vi "Main.vi"(11 "Module Admin":refnum<class "Delacor_lib_QMH_Module Admin.lvclass">) -> ()   [LabVIEW 2016, in "Lab Streaming Layer.lvlib"]
doc: "This template is based off of the Queued Message Handler design pattern and the Queued Message Handler project template that ships with LabVIEW.\n\nThe main difference is that the queue is private to this module and communication between modules is performed via Broadcast and Request events.\n\nRequest events are wrapped in public API methods and are handled in the Event Handling Loop (EHL) of this VI. Any module can register for Broadcast events sent by this module. The EHL generates messages based on user interface actions.\n\nThe Message Handling Loop (MHL) processes messages generated by the EHL, or by other messages. The messages are string values, so new messages can be added easily to the Message Cases case structure in the MHL. Each message cluster can also provide an optional value for Message Data, which is a variant that can be converted to whatever message-specific data is required.\n_____\nBased on DQMH Project Template 7.0.0.1280."
uses:
  Lab Streaming Layer.lvlib
  <vilib>/Delacor/Delacor QMH/Libraries/Module Admin_class/Delacor_lib_QMH_Module Admin.lvclass
  Module Data--cluster.ctl
  Custom Controls/lsl_channel_format.ctl
  Custom Controls/lsl_outlet.ctl
  Custom Controls/lsl_streaminfo.ctl
  Custom Controls/lsl_xml_ptr.ctl
  <vilib>/Delacor/Delacor QMH/Libraries/Message Queue_class/Delacor_lib_QMH_Message Queue.lvclass/Delacor_lib_QMH_Message Queue.ctl
  Stop Argument--cluster.ctl
  <vilib>/Delacor/Delacor QMH/Libraries/Module Admin_class/Delacor_lib_QMH_Module Admin.lvclass/Delacor_lib_QMH_Module Admin.ctl
  Init LSL Metadata Argument--cluster.ctl
  Stop Stream Argument--cluster.ctl
  LSL Stream Data Argument--cluster.ctl
  Acquisition/WiBCI16T_Data.ctl
  Acquisition/WiBCI16T_Status.ctl
  Acquisition/Reg_Map.ctl
  Get Listeners count Argument--cluster.ctl
  Get Listeners count (Reply Payload)--cluster.ctl
  KeyBoard Trigger Argument--cluster.ctl
  <vilib>/Utility/miscctls.llb/LVPointTypeDef.ctl
  <vilib>/Delacor/Delacor QMH/Libraries/Message Queue_class/Delacor_lib_QMH_Enqueue Message (Single).vi
  <vilib>/Delacor/Delacor QMH/Libraries/Module Admin_class/Delacor_lib_QMH_Get External Launch.vi
  <vilib>/Delacor/Delacor QMH/Libraries/Message Queue_class/Delacor_lib_QMH_Message Queue.lvclass
  Settings Editor/Settings Editor.lvlib
  Acquisition/Acquisition.lvlib
panel:
  out "error out 2":errorcluster
  out "error out":errorcluster
  out "Status":string
  in  "Simulate MHL Error":bool
  in  "Simulate EHL Error":bool
  # "This template is for the DQMH framework. See the block diagram for more information on how to use this template."
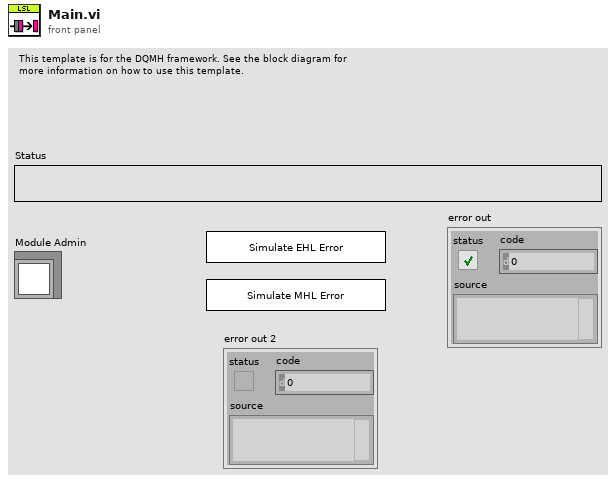
[diagram p1: front panel]
types:
  T1 = typedef "Settings Editor.lvlib/Broadcast Events--cluster.ctl" = cluster{"Module Did Init":refnum<user-event>, "Status Updated":refnum<user-event>, "Error Reported":refnum<user-event>, "Module Did Stop":refnum<user-event>, "Update Module Execution Status":refnum<user-event>, "Application Settings Updated":refnum<user-event>}
  T2 = typedef "Lab Streaming Layer.lvlib/Request Events--cluster.ctl" = cluster{"Stop Module":refnum<user-event>, "Show Panel":refnum<user-event>, "Hide Panel":refnum<user-event>, "Get Module Execution Status":refnum<user-event>, "Show Diagram":refnum<user-event>, "Init LSL Metadata":refnum<user-event>, "Stop Stream":refnum<user-event>, "LSL Stream Data":refnum<user-event>, "Get Listeners count":refnum<user-event>, "KeyBoard Trigger":refnum<user-event>}
  T3 = typedef "Lab Streaming Layer.lvlib/Module Data--cluster.ctl" = cluster{"Status":string, "LSL Streaming":bool, "channel_format":T4, "outlet":T5, "streaminfo":T6, "xml_ptr":T7, "LSL Listeners":i32, "LSL Listeners Query Counter":i32, "Data Chunk ":cluster{"counter":u8, "Data":dbl[][]}, "Ch En Map":bool[], "outlet mark":T5, "streaminfo mark":T6, "xml_ptr mark":T7}
  T4 = typedef "Lab Streaming Layer.lvlib/lsl_channel_format.ctl" = u32
  T5 = typedef "Lab Streaming Layer.lvlib/lsl_outlet.ctl" = u64
  T6 = typedef "Lab Streaming Layer.lvlib/lsl_streaminfo.ctl" = u64
  T7 = typedef "Lab Streaming Layer.lvlib/lsl_xml_ptr.ctl" = u64
  T8 = enum32{"invalid lock state", "Not Locked", "Locked (No Password)", "Password-protected"}
  T9 = typedef "Lab Streaming Layer.lvlib/Stop Argument--cluster.ctl" = cluster{"Origin":string, "Exit via Stop Module Req?":bool, "Wait for Module to stop?":bool}
  T10 = typedef "Lab Streaming Layer.lvlib/Init LSL Metadata Argument--cluster.ctl" = cluster{"Boolean":bool}
  T11 = typedef "Lab Streaming Layer.lvlib/Stop Stream Argument--cluster.ctl" = cluster{"Boolean":bool}
  T12 = typedef "Lab Streaming Layer.lvlib/LSL Stream Data Argument--cluster.ctl" = cluster{"WiBCI16T Data":T13}
  T13 = typedef "Acquisition.lvlib/WiBCI16T_Data.ctl" = cluster{"EEG Ch 1":dbl, "EEG Ch 2":dbl, "EEG Ch 3":dbl, "EEG Ch 4":dbl, "EEG Ch 5":dbl, "EEG Ch 6":dbl, "EEG Ch 7":dbl, "EEG Ch 8":dbl, "EEG Ch 9":dbl, "EEG Ch 10":dbl, "EEG Ch 11":dbl, "EEG Ch 12":dbl, "EEG Ch 13":dbl, "EEG Ch 14":dbl, "EEG Ch 15":dbl, "EEG Ch 16":dbl, "X-Accel":i16, "Y-Accel":i16, "Z-Accel":i16, "X-Gyro":i16, "Y-Gyro":i16, "Z-Gyro":i16, "Timer":u32, "Packet ID":u32, "HW Trig1":u8, "SW Trig1":i8, "HW Trig2":u8, "SW Trig2":i8, "WiBCI Status":T14, "Reg Map":T15}
  T14 = typedef "Acquisition.lvlib/WiBCI16T_Status.ctl" = cluster{"Mode Byte":u8, "Ch Config":u8, "Ch Ref Map":u16, "Ch Enable Map":u16, "Temperature":sgl, "Battery":u8, "Version":string}
  T15 = typedef "Acquisition.lvlib/Reg_Map.ctl" = cluster{"ADS1":u8[], "ADS2":u8[]}
  T16 = typedef "Lab Streaming Layer.lvlib/Get Listeners count Argument--cluster.ctl" = cluster{"Wait Notifier":refnum<notifier>, "wait for reply":bool}
  T17 = typedef "Lab Streaming Layer.lvlib/KeyBoard Trigger Argument--cluster.ctl" = cluster{"Keyboard Trig":i16}
  T18 = typedef "LVPointTypeDef.ctl" = cluster{"Horizontal":i16, "Vertical":i16}
  T19 = enum32{"Invalid", "Standard", "Closed", "Hidden", "Minimized", "Maximized"}
  T20 = typedef "Lab Streaming Layer.lvlib/Get Listeners count (Reply Payload)--cluster.ctl" = cluster{"Listeners":i32, "error":errorcluster}
  T21 = typedef "Settings Editor.lvlib/Update Application Settings (Reply Payload)--cluster.ctl" = cluster{"Settings":T22, "error":errorcluster}
  T22 = typedef "Settings Editor.lvlib/Settings--cluster.ctl" = cluster{"Signal Type":T23, "Calibration Array":T24[], "Log File Base Path":path, "EEG Channels":T25, "Soft Trig enum":enum16{"Disable Soft Trigger", "Enable Soft Trigger"}, "Montage selection":cluster{"Montages Ref":refnum<vi>, "Selected Montage Number":u8, "Montages Names":string[]}, "LSL En enum":enum16{"LSL Disabled", "LSL Enabled"}}
  T23 = typedef "Acquisition.lvlib/Signal Type--enum.ctl" = enum16{"Sine Wave", "Square with Noise"}
  T24 = typedef "Acquisition.lvlib/Calibration Values--cluster.ctl" = cluster{"Slope":dbl, "Offset":dbl}
  T25 = typedef "CML Shared.lvlib/EEG Channel Settings.ctl" = cluster{"16 EEG Channels":cluster{"Channel Name":string, "Channel No":u8, "Channel Enabled":bool, "Channel Referenced":bool}[], "Gain":u8}
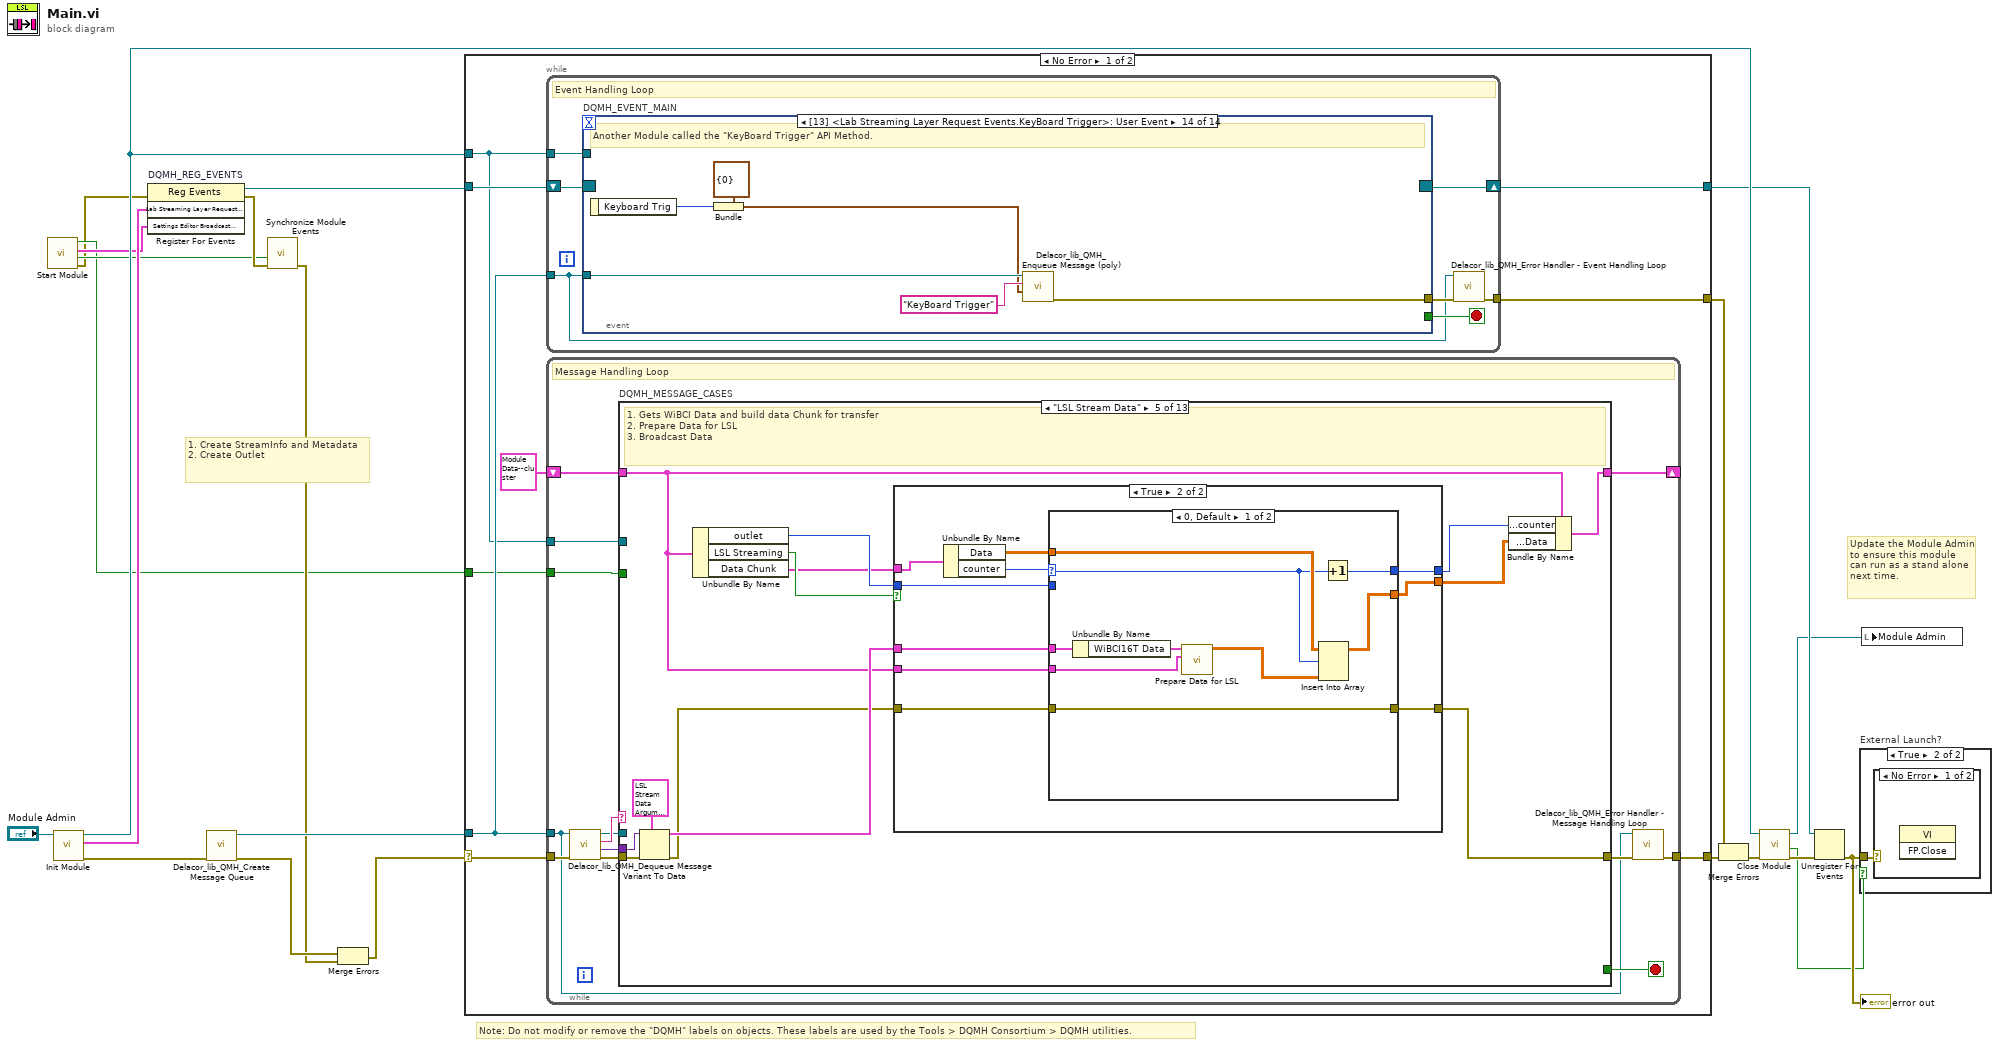
[diagram p0: block diagram]
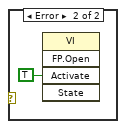
[diagram p3: hidden frame]
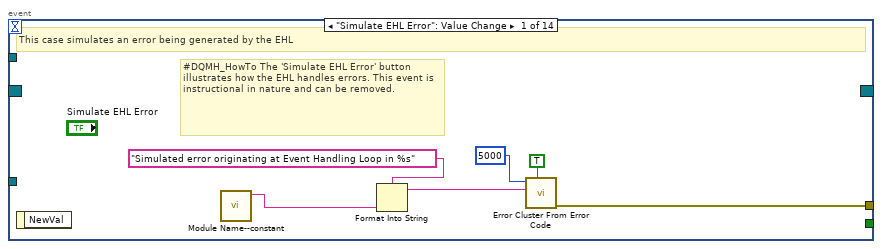
[diagram p4: hidden frame]
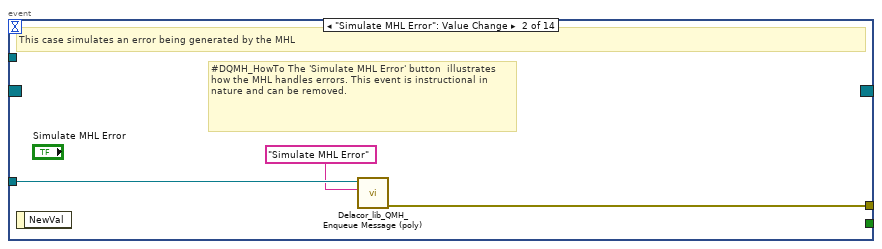
[diagram p5: hidden frame]
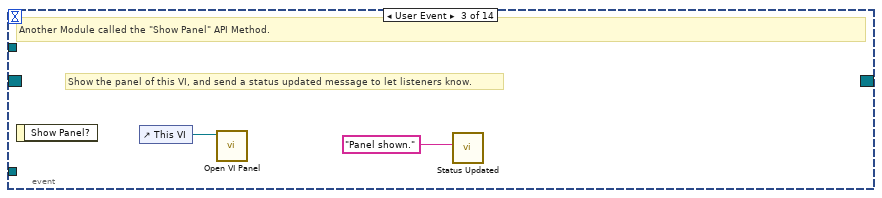
[diagram p6: hidden frame]
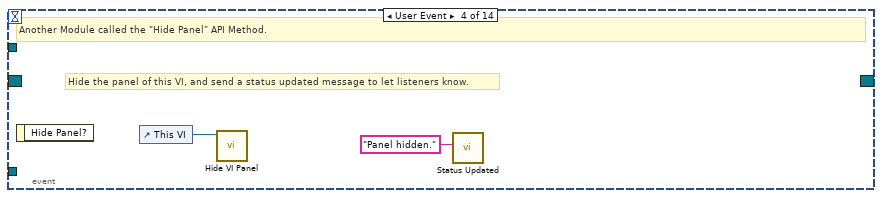
[diagram p7: hidden frame]
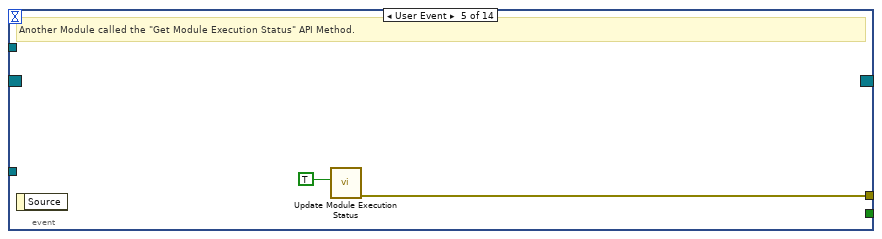
[diagram p8: hidden frame]
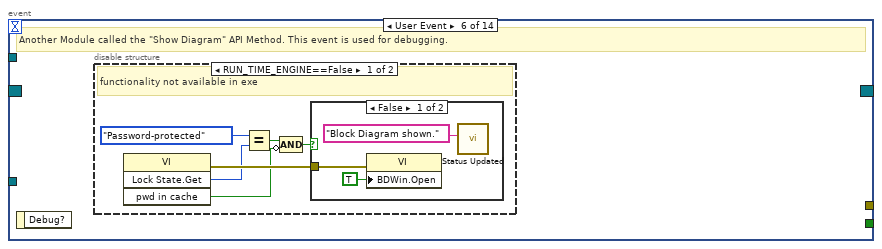
[diagram p9: hidden frame]
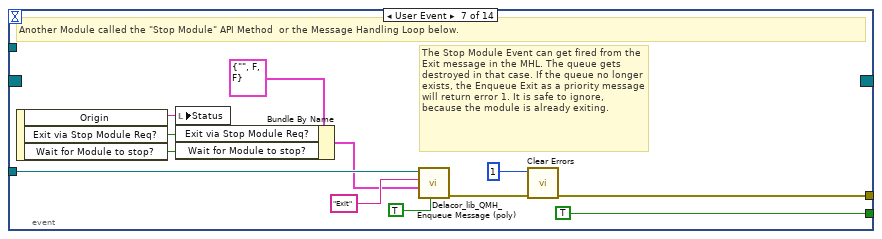
[diagram p12: hidden frame]
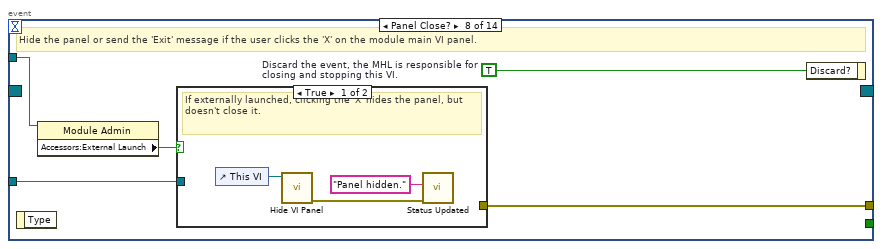
[diagram p13: hidden frame]
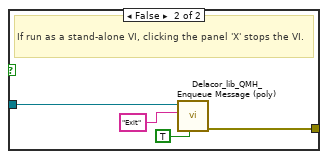
[diagram p14: hidden frame]
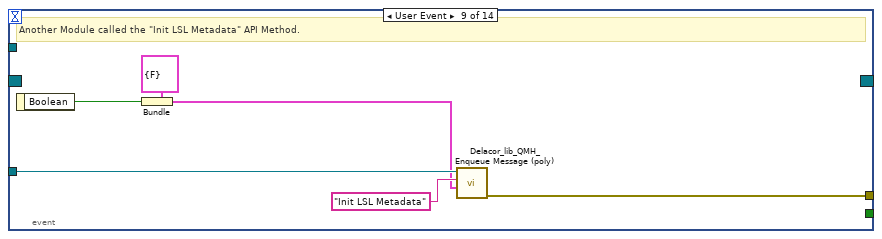
[diagram p15: hidden frame]
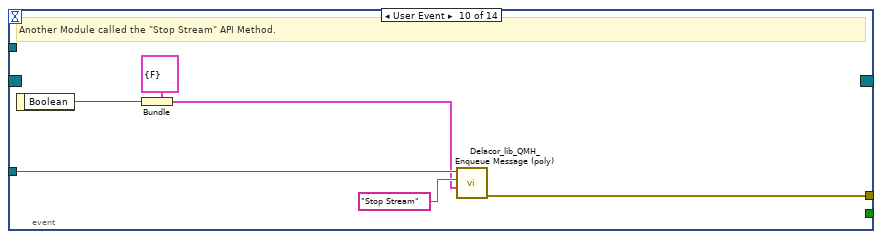
[diagram p16: hidden frame]
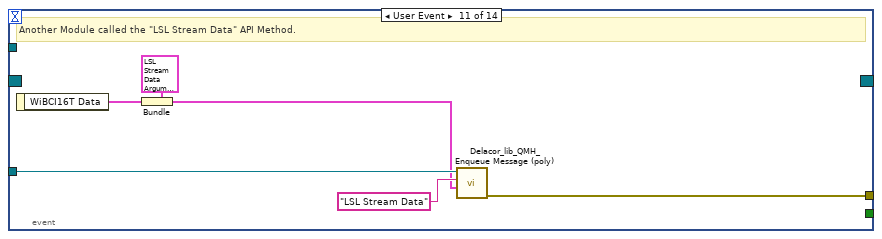
[diagram p17: hidden frame]
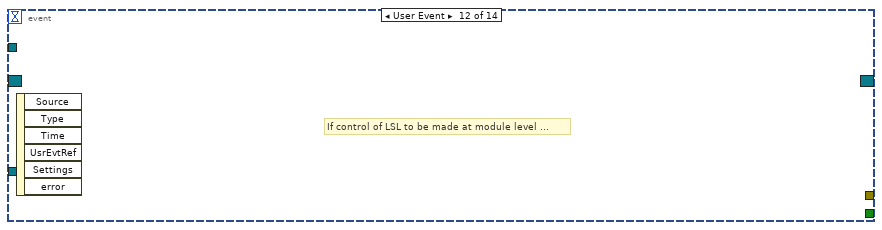
[diagram p18: hidden frame]
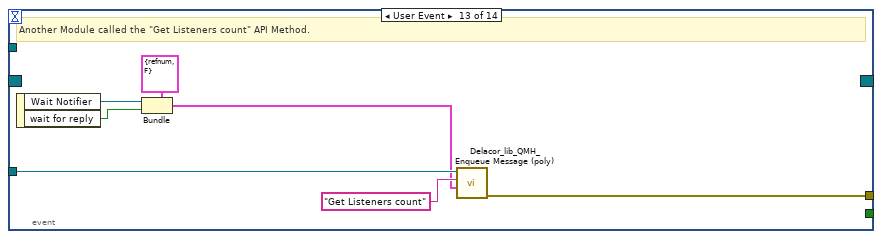
[diagram p19: hidden frame]
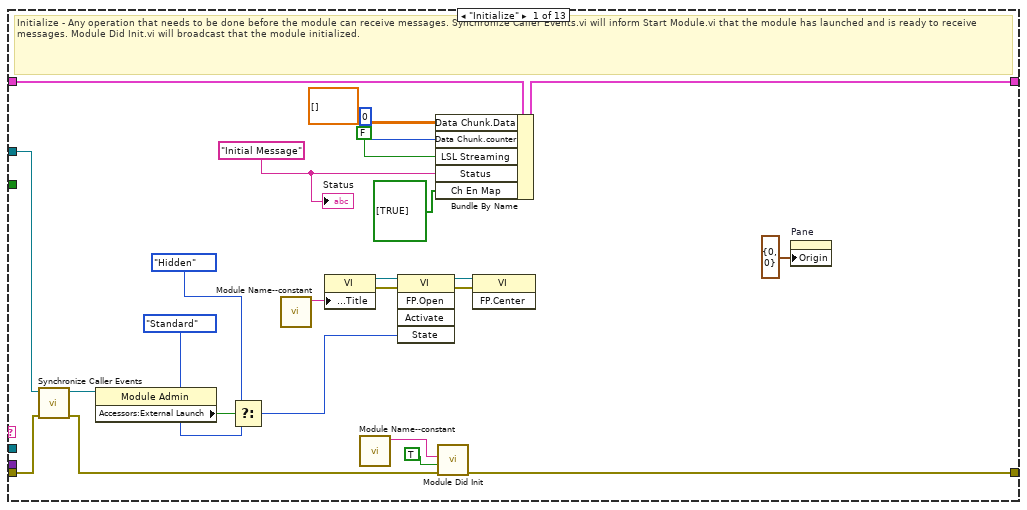
[diagram p20: hidden frame]
diagram:
  # "1. Create StreamInfo and Metadata\n2. Create Outlet"
  # "Note: Do not modify or remove the \"DQMH\" labels on objects. These labels are used by the Tools > DQMH Consortium > DQMH utilities."
  # "Update the Module Admin to ensure this module can run as a stand alone next time."
  n1 = call "Start Module.vi"() -> ("error out"=w1:errorcluster, "Wait for Event Sync?"=w3:bool, "Settings Editor Broadcast Events"=w6:T1, "Module Was Already Running?"=w2:bool)  [unwired: 8 in]
  n2 = call "Init Module.vi"("Singleton Module Admin in"="Module Admin") -> ("error out"=w21:errorcluster, "Lab Streaming Layer Request Events"=w11:T2, "Singleton Module Admin out"=w14:refnum<class "Delacor_lib_QMH_Module Admin.lvclass">)  [unwired: 8 in]
  n3 = register-events "DQMH_REG_EVENTS"(error in=w1, w11, w6) -> (reference out=w12:refnum<event-registration>, error out=w5:errorcluster)  [unwired: 1 in]
  n4 = call <vilib>:"Delacor_lib_QMH_Create Message Queue.vi"("error in"=w21) -> ("error out"=w16:errorcluster, "Message Queue"=w10:refnum<class "Delacor_lib_QMH_Message Queue.lvclass">)  [unwired: 9 in]
  n5 = call "Synchronize Module Events.vi"("error in (no error)"=w5, "Wait for Event Sync?"=w3) -> ("error out"=w4:errorcluster)  [unwired: 9 in]
  n6 = Merge Errors(w16, w4) -> (w15:errorcluster)
  n7 = case shown="No Error" w15 {
    selector: w15 -> [w29 w392]
    tunnel: [w31 w391] -> w22
    tunnel: [w28 w390] -> w13
    tunnel: w12 -> [w26 w390]
    tunnel: w10 -> [w25 w385]
    tunnel: [w30 _] -> w19
    tunnel: w14 -> [w24 w386]
    tunnel: w2 -> [w23 _]
    frame No Error {
      n8 = while {
        tunnel: w25 -> [w32]
        shift-right: [w35] -> w28
        shift-left: w26 -> [w36]
        tunnel: [w37] -> w30
        tunnel: w24 -> [w33]
        stop <- w34 stop-if-true
        # "Event Handling Loop"
        n9 = event "DQMH_EVENT_MAIN" shown="[13] <Lab Streaming Layer Request Events.KeyBoard Trigger>: User Event" {
          selector: w36 -> [_ _ _ _ _ _ _ _ _ _ _ _ _ _]
          dyn-events: [_ _ _ _ _ _ _ _ _ _ _ _ _ _] -> w35
          timeout: _ -> [_ _ _ _ _ _ _ _ _ _ _ _ _ _]
          tunnel: [_ _ _ _ _ _ TRUE ("Discard?") _ _ _ _ _ _ _] -> w34
          tunnel: w32 -> [_ w46 _ _ _ _ w70 w77 w92 w98 w104 _ w111 w117]
          tunnel: [w44 w47 _ _ w53 _ w73 w79 w87 w93 w99 _ w105 w112] -> w38
          tunnel: w33 -> [_ _ _ _ _ _ _ w76 _ _ _ _ _ _]
          event "Simulate EHL Error": Value Change {
            # "#DQMH_HowTo The 'Simulate EHL Error' button  illustrates how the EHL handles errors. This event is instructional in nature and can be removed."
            # "This case simulates an error being generated by the EHL"
            n10 = event-data() -> ()  [unwired: 1 in, 1 out]
            n11 = call "Module Name--constant.vi"() -> ("Module Name"=w41:string)  [unwired: 11 in]
            n12 = Format Into String(format string="Simulated error originating at Event Handling Loop in %s", w41) -> (resulting string=w42:string)  [unwired: 2 in, 1 out]
            n13 = call <vilib>:"Error Cluster From Error Code.vi"("show call chain? (False)"=TRUE, "error message (\"\")"=w42, "error code (0)"=5000) -> ("error out"=w44:errorcluster)  [unwired: 6 in]
          }
          event "Simulate MHL Error": Value Change {
            # "#DQMH_HowTo The 'Simulate MHL Error' button  illustrates how the MHL handles errors. This event is instructional in nature and can be removed."
            # "This case simulates an error being generated by the MHL"
            n14 = event-data() -> ()  [unwired: 1 in, 1 out]
            n15 = call-poly <vilib>:"Delacor_lib_QMH_Enqueue Message (poly).vi"("Message"="Simulate MHL Error", "Message Queue in"=w46) -> ("error out"=w47:errorcluster)  [unwired: 8 in, 1 out]
          }
          event User Event {
            # "Show the panel of this VI, and send a status updated message to let listeners know."
            # "Another Module called the \"Show Panel\" API Method."
            n16 = event-data() -> ()  [unwired: 1 in, 1 out]
            n17 = control-ref of="This VI"() -> (w49:refnum<vi>)
            n18 = call "Open VI Panel.vi"("VI"=w49) -> ()  [unwired: 10 in, 1 out]
            n19 = call "Status Updated.vi"("Status"="Panel shown." ("format string")) -> ()  [unwired: 10 in, 1 out]
          }
          event User Event {
            # "Hide the panel of this VI, and send a status updated message to let listeners know."
            # "Another Module called the \"Hide Panel\" API Method."
            n20 = event-data() -> ()  [unwired: 1 in, 1 out]
            n21 = control-ref of="This VI"() -> (w51:refnum<vi>)
            n22 = call "Hide VI Panel.vi"("VI"=w51) -> ()  [unwired: 10 in, 1 out]
            n23 = call "Status Updated.vi"("Status"="Panel hidden." ("format string")) -> ()  [unwired: 10 in, 1 out]
          }
          event User Event {
            # "Another Module called the \"Get Module Execution Status\" API Method."
            n24 = event-data() -> ()  [unwired: 1 in, 1 out]
            n25 = call "Update Module Execution Status.vi"("Running?"=TRUE) -> ("error out"=w53:errorcluster)  [unwired: 10 in]
          }
          event User Event {
            # "Another Module called the \"Show Diagram\" API Method. This event is used for debugging."
            n26 = event-data() -> ()  [unwired: 1 in, 1 out]
            n27 = disable-structure shown="RUN_TIME_ENGINE==False" {
              frame condition #0 (active) {
                # "functionality not available in exe"
                n28 = invoke class="VI" method="Lock State.Get"() -> (error out=w59:errorcluster, "Get Lock State"=w58:T8, "pwd in cache"=w55:bool)  [unwired: 4 in, 1 out]
                n29 = Equal?(x=T8."Password-protected", y=w58) -> (x = y?=w56:bool)
                n30 = Compound Arithmetic op=AND(w56, invert w55) -> (w54:bool)
                n31 = case shown="False" w54 {
                  tunnel: w59 -> [w62 _]
                  frame False {
                    n32 = property class="VI"(error in=w62, "BDWin.Open"=TRUE ("Block Diagram Window:Open")) -> ()  [unwired: 1 in, 2 out]
                    n33 = call "Status Updated.vi"("Status"="Block Diagram shown." ("format string")) -> ()  [unwired: 10 in, 1 out]
                  }
                  frame True {
                    # "Password-protected VI, and the password is not in the cache. Do not show the diagram."
                  }
                }
              }
              frame condition #1 {
              }
            }
          }
          event User Event {
            # "The Stop Module Event can get fired from the Exit message in the MHL. The queue gets destroyed in that case. If the queue no longer exists, the Enqueue Exit as a priority message will return error 1. It is safe to ignore, because the module is already exiting."
            # "Another Module called the \"Stop Module\" API Method  or the Message Handling Loop below."
            n34 = event-data() -> ("Origin"=w69:string, "Exit via Stop Module Req?"=w65:bool, "Wait for Module to stop?"=w64:bool)  [unwired: 1 in]
            n35 = local write "Status"(w69) -> ()
            n36 = Bundle By Name(cluster=T9 {"Origin"="", "Exit via Stop Module Req?"=FALSE, "Wait for Module to stop?"=FALSE} ("Stop Argument"), "Exit via Stop Module Req?"=w65, "Wait for Module to stop?"=w64) -> (w63:T9)
            n37 = call-poly <vilib>:"Delacor_lib_QMH_Enqueue Message (poly).vi"("Priority Message? (F)"=TRUE, "Message Data"=w63, "Message"="Exit", "Message Queue in"=w70) -> ("error out"=w74:errorcluster)  [unwired: 6 in, 1 out]
            n38 = call <vilib>:"Clear Errors.vi"("error in (no error)"=w74, "specific error code to clear (0: all)"=1) -> ("error out"=w73:errorcluster)  [unwired: 4 in, 1 out]
          }
          event Panel Close? {
            w78 = TRUE  # Discard the event, the MHL is responsible for closing and stopping this VI.
            # "Hide the panel or send the 'Exit' message if the user clicks the 'X' on the module main VI panel."
            n39 = event-data() -> ()  [unwired: 1 in, 1 out]
            n40 = property class="Module Admin"(reference=w76) -> ("Accessors:External Launch"=w75:bool)  [unwired: 1 in, 2 out]
            n41 = case shown="True" w75 {
              tunnel: w77 -> [_ w85]
              tunnel: [_ w86] -> w79
              frame True {
                # "If externally launched, clicking the 'X' hides the panel, but doesn't close it."
                n42 = control-ref of="This VI"() -> (w82:refnum<vi>)
                n43 = call "Hide VI Panel.vi"("VI"=w82) -> ("error out"=w80:errorcluster)  [unwired: 10 in]
                n44 = call "Status Updated.vi"("error in"=w80, "Status"="Panel hidden." ("format string")) -> ()  [unwired: 9 in, 1 out]
              }
              frame False {
                # "If run as a stand-alone VI, clicking the panel 'X' stops the VI."
                n45 = call-poly <vilib>:"Delacor_lib_QMH_Enqueue Message (poly).vi"("Priority Message? (F)"=TRUE, "Message"="Exit", "Message Queue in"=w85) -> ("error out"=w86:errorcluster)  [unwired: 7 in, 1 out]
              }
            }
            n46 = event-data("Discard?"=w78) -> ()  [unwired: 1 in, 1 out]
          }
          event User Event {
            # "Another Module called the \"Init LSL Metadata\" API Method."
            n47 = event-data() -> ("Boolean"=w88:bool)  [unwired: 1 in]
            n48 = Bundle(cluster=T10 {"Boolean"=FALSE} ("Init LSL Metadata Argument"), "Boolean"=w88) -> (w89:T10)
            n49 = call-poly <vilib>:"Delacor_lib_QMH_Enqueue Message (poly).vi"("Message Data"=w89, "Message"="Init LSL Metadata", "Message Queue in"=w92) -> ("error out"=w87:errorcluster)  [unwired: 7 in, 1 out]
          }
          event User Event {
            # "Another Module called the \"Stop Stream\" API Method."
            n50 = event-data() -> ("Boolean"=w94:bool)  [unwired: 1 in]
            n51 = Bundle(cluster=T11 {"Boolean"=FALSE} ("Stop Stream Argument"), "Boolean"=w94) -> (w95:T11)
            n52 = call-poly <vilib>:"Delacor_lib_QMH_Enqueue Message (poly).vi"("Message Data"=w95, "Message"="Stop Stream", "Message Queue in"=w98) -> ("error out"=w93:errorcluster)  [unwired: 7 in, 1 out]
          }
          event User Event {
            # "Another Module called the \"LSL Stream Data\" API Method."
            n53 = event-data() -> ("WiBCI16T Data"=w100:T13)  [unwired: 1 in]
            n54 = Bundle(cluster=T12 {"WiBCI16T Data"={"EEG Ch 1"=0.0, "EEG Ch 2"=0.0, "EEG Ch 3"=0.0, "EEG Ch 4"=0.0, "EEG Ch 5"=0.0, "EEG Ch 6"=0.0, "EEG Ch 7"=0.0, "EEG Ch 8"=0.0, "EEG Ch 9"=0.0, "EEG Ch 10"=0.0, "EEG Ch 11"=0.0, "EEG Ch 12"=0.0, "EEG Ch 13"=0.0, "EEG Ch 14"=0.0, "EEG Ch 15"=0.0, "EEG Ch 16"=0.0, "X-Accel"=0, "Y-Accel"=0, "Z-Accel"=0, "X-Gyro"=0, "Y-Gyro"=0, "Z-Gyro"=0, "Timer"=0, "Packet ID"=0, "HW Trig1"=0, "SW Trig1"=0, "HW Trig2"=0, "SW Trig2"=0, "WiBCI Status"={"Mode Byte"=0, "Ch Config"=0, "Ch Ref Map"=0, "Ch Enable Map"=0, "Temperature"=0.0, "Battery"=0, "Version"=""}, "Reg Map"={"ADS1"=[], "ADS2"=[]}}} ("LSL Stream Data Argument"), "WiBCI16T Data"=w100) -> (w101:T12)
            n55 = call-poly <vilib>:"Delacor_lib_QMH_Enqueue Message (poly).vi"("Message Data"=w101, "Message"="LSL Stream Data", "Message Queue in"=w104) -> ("error out"=w99:errorcluster)  [unwired: 7 in, 1 out]
          }
          event User Event {
            # "If control of LSL to be made at module level ..."
            n56 = event-data() -> ()  [unwired: 1 in, 6 out]
          }
          event User Event {
            # "Another Module called the \"Get Listeners count\" API Method."
            n57 = event-data() -> ("Wait Notifier"=w107:refnum<notifier>, "wait for reply"=w106:bool)  [unwired: 1 in]
            n58 = Bundle(cluster=T16 {"Wait Notifier"=refnum, "wait for reply"=FALSE} ("Get Listeners count Argument"), "Wait Notifier"=w107, "wait for reply"=w106) -> (w108:T16)
            n59 = call-poly <vilib>:"Delacor_lib_QMH_Enqueue Message (poly).vi"("Message Data"=w108, "Message"="Get Listeners count", "Message Queue in"=w111) -> ("error out"=w105:errorcluster)  [unwired: 7 in, 1 out]
          }
          event User Event {
            # "Another Module called the \"KeyBoard Trigger\" API Method."
            n60 = event-data() -> ("Keyboard Trig"=w113:i16)  [unwired: 1 in]
            n61 = Bundle(cluster=T17 {"Keyboard Trig"=0} ("KeyBoard Trigger Argument"), "Keyboard Trig"=w113) -> (w114:T17)
            n62 = call-poly <vilib>:"Delacor_lib_QMH_Enqueue Message (poly).vi"("Message Data"=w114, "Message"="KeyBoard Trigger", "Message Queue in"=w117) -> ("error out"=w112:errorcluster)  [unwired: 7 in, 1 out]
          }
        }
        n63 = call-dynamic "Delacor_lib_QMH_Error Handler - Event Handling Loop.vi"("error in"=w38, "Message Queue in"=w32) -> ("dup error in"=w37:errorcluster)  [unwired: 8 in, 1 out]
      }
      n64 = while {
        tunnel: w25 -> [w119]
        shift-right: [w125] -> _
        shift-left: T3 {"Status"="", "LSL Streaming"=FALSE, "channel_format"=1, "outlet"=0, "streaminfo"=0, "xml_ptr"=0, "LSL Listeners"=0, "LSL Listeners Query Counter"=0, "Data Chunk "={"counter"=0, "Data"=[]}, "Ch En Map"=[], "outlet mark"=0, "streaminfo mark"=0, "xml_ptr mark"=0} ("Data Cluster") -> [w126]
        tunnel: w29 -> [w129]
        tunnel: [w127] -> w31
        tunnel: w24 -> [w120]
        tunnel: w23 -> [w118]
        stop <- w124 stop-if-true
        # "Message Handling Loop"
        n65 = call-dynamic "Delacor_lib_QMH_Dequeue Message.vi"("error in"=w129, "Message Queue in"=w119) -> ("error out"=w128:errorcluster, "Message Data"=w122:variant, "Message"=w123:string, "Message Queue out"=w121:refnum<class "Delacor_lib_QMH_Message Queue.lvclass">)  [unwired: 6 in]
        n66 = case "DQMH_MESSAGE_CASES" shown="\"LSL Stream Data\"" w123 {
          selector: w123 -> [_ _ _ _ _ _ _ _ _ _ _ _ w380]
          tunnel: w121 -> [_ _ _ _ _ _ _ _ _ _ w342 w366 _]
          tunnel: w128 -> [w152 w156 w165 w218 w249 w300 w318 w327 w329 w338 w349 w372 w383]
          tunnel: [w150 w156 w157 w209 w243 w292 w309 w326 w329 w337 w345 w367 w384] -> w130
          tunnel: w126 -> [w141 w155 w159 w214 w237 w291 w314 w325 w328 w335 w344 w365 w381]
          tunnel: [w140 w155 w158 w213 w240 w291 w314 w325 w328 w335 w344 w365 w381] -> w125
          tunnel: [_ _ _ _ _ _ _ _ _ _ _ w364 _] -> w124
          tunnel: w122 -> [_ _ w164 w217 w248 w299 w317 _ _ _ w343 w363 _]
          tunnel: w120 -> [w142 _ _ _ _ _ _ _ _ _ w341 w358 _]
          tunnel: w118 -> [_ _ _ _ _ _ _ _ _ _ _ w356 _]
          frame "Initialize" {
            w136 = "Initial Message" ("Initial Message")
            # "Initialize - Any operation that needs to be done before the module can receive messages. Synchronize Caller Events.vi will inform Start Module.vi that the module has launched and is ready to receive messages. Module Did Init.vi will broadcast that the module initialized."
            n67 = call "Synchronize Caller Events.vi"("error in"=w152, "Singleton Module Admin in"=w142) -> ("error out"=w151:errorcluster, "Singleton Module Admin out"=w137:refnum<class "Delacor_lib_QMH_Module Admin.lvclass">)  [unwired: 8 in]
            n68 = property class="Module Admin"(reference=w137) -> ("Accessors:External Launch"=w146:bool)  [unwired: 1 in, 2 out]
            n69 = Select(t=T19."Hidden" ("State"), s=w146, f=T19."Standard" ("State")) -> (s? t:f=w143:T19)
            n70 = call "Module Name--constant.vi"() -> ("Module Name"=w149:string)  [unwired: 11 in]
            n71 = property class="VI"("Front Panel.Title"=w149) -> (reference out=w148:refnum<vi>, error out=w154:errorcluster)  [unwired: 2 in]
            n72 = call "Module Name--constant.vi"() -> ("Module Name"=w138:string)  [unwired: 11 in]
            n73 = invoke class="VI" method="FP.Open"(reference=w148, error in=w154, "State"=w143) -> (reference out=w147:refnum<vi>, error out=w153:errorcluster)  [unwired: 2 in, 3 out]
            n74 = Bundle By Name(cluster=w141, "Data Chunk.Data"=dbl[][] [] ("Data Chunk .Data"), "Data Chunk.counter"=u8 0 ("Data Chunk .counter"), "LSL Streaming"=FALSE, "Status"=w136, "Ch En Map"=bool[] [TRUE]) -> (w140:T3)
            n75 = call "Module Did Init.vi"("error in"=w151, "Initialized?"=TRUE, "Origin"=w138) -> ("error out"=w150:errorcluster)  [unwired: 8 in]
            n76 = invoke class="VI" method="FP.Center"(reference=w147, error in=w153) -> ()  [unwired: 1 in, 3 out]
            n77 = property on="Pane" class="Pane"("Origin"=T18 {"Horizontal"=0, "Vertical"=0}) -> ()  [unwired: 2 in, 2 out]
            "Status" <- w136
          }
          frame "---Module Specific---" {
            # "Separator -- The following cases handle messages specific to this Module."
          }
          frame "Init LSL Metadata" {
            # "Initialize LSL metadata for Broadcasting of data"
            n78 = Variant To Data(error in=w165, type=T10 {"Boolean"=FALSE} ("Init LSL Metadata Argument"), Variant=w164) -> (error out=w160:errorcluster)  [unwired: 1 out]
            n79 = call "Update Application Settings.vi"("error in"=w160) -> ("error out"=w162:errorcluster, "Reply Payload"=w161:T21)  [unwired: 8 in, 1 out]
            n80 = case shown="No Error" w162 {
              selector: w162 -> [w167 w205]
              tunnel: w161 -> [w172 _]
              tunnel: w159 -> [w168 w206]
              tunnel: [w171 w206] -> w158
              tunnel: [w170 w205] -> w157
              frame No Error {
                n81 = call "Get SSID.vi"() -> ("Amplifier Connected ?"=w166:bool, "SSID"=w169:string)  [unwired: 10 in]
                n82 = case shown="True" w166 {
                  tunnel: w172 -> [_ w204]
                  tunnel: [w174 w195] -> w171
                  tunnel: [w173 w175] -> w170
                  tunnel: w169 -> [_ w193]
                  tunnel: w168 -> [w174 w191]
                  tunnel: w167 -> [w173 w190]
                  frame False {
                    # "Not a Amplifier WiFI AP\nNo need to start a stream"
                  }
                  frame True {
                    w183 = T4 2 items=["cft_float32"=1, "cft_double64"=2, "cft_string"=3, "cft_int32"=4, "cft_int16"=5, "cft_int8"=6, "cft_int64"=7, "cft_undefined"=0] ("channel_format")
                    w203 = T4 2 items=["cft_float32"=1, "cft_double64"=2, "cft_string"=3, "cft_int32"=4, "cft_int16"=5, "cft_int8"=6, "cft_int64"=7, "cft_undefined"=0] ("channel_format")
                    # "2."
                    # "1."
                    n83 = call "Get En and Ref Channels.vi"("Reply Payload"=w204) -> ("Ch Names"=w186:string[], "Ch En Map"=w187:bool[])  [unwired: 7 in, 2 out]
                    n84 = Array Size(array=w186) -> (size(s)=w200:i32)
                    n85 = call "lsl create streaminfo.vi"("source_id"=w193, "channel_format"=w203, "samplingrate"=250.0, "error in (no error)"=w190, "channel_count"=w200, "type"="EEG", "name"=w193) -> ("error out"=w199:errorcluster, "streaminfo"=w197:T6)  [unwired: 3 in]
                    n86 = call "Set MetaData for Stream.vi"("error in"=w199, "Ch Names"=w186, "streaminfo"=w197) -> ("error out"=w198:errorcluster)  [unwired: 8 in]
                    n87 = call "lsl create streaminfo.vi"("source_id"="WiBCI16T-V0001-0001_Markers", "channel_format"=w183, "channel_count"=1, "type"="Marker", "name"="My EEG Device Markers") -> ("error out"=w184:errorcluster, "streaminfo"=w179:T6)  [unwired: 5 in]
                    n88 = call "lsl create outlet.vi"("error in (no error)"=w198, "streaminfo"=w197) -> ("error out"=w177:errorcluster, "outlet"=w196:T5)  [unwired: 8 in]
                    n89 = call "lsl create outlet.vi"("error in (no error)"=w184, "streaminfo"=w179) -> ("error out"=w176:errorcluster, "outlet"=w178:T5)  [unwired: 8 in]
                    "error out 2" <- w176
                    n90 = Merge Errors(w177, w176) -> (w175:errorcluster)
                    n91 = Bundle By Name(cluster=w191, "Ch En Map"=w187, "Data Chunk.Data"=dbl[][] [] ("Data Chunk .Data"), "Data Chunk.counter"=u8 0 ("Data Chunk .counter"), "Status"="Start Steam ...", "LSL Streaming"=TRUE, "streaminfo"=w197, "outlet"=w196, "streaminfo mark"=w179, "outlet mark"=w178) -> (w195:T3)
                  }
                }
              }
              frame Error {
              }
            }
          }
          frame "Stop Stream" {
            # "Stops the LSL data broadcast."
            n92 = Variant To Data(error in=w218, type=T11 {"Boolean"=FALSE} ("Stop Stream Argument"), Variant=w217) -> (error out=w211:errorcluster)  [unwired: 1 out]
            n93 = Unbundle By Name(w214) -> ("LSL Streaming"=w215:bool, "outlet"=w212:T5, "streaminfo"=w210:T6, "outlet mark"=w208:T5, "streaminfo mark"=w207:T6)
            n94 = case shown="True" w215 {
              tunnel: w214 -> [w220 w235]
              tunnel: [w220 w234] -> w213
              tunnel: w212 -> [_ w232]
              tunnel: w211 -> [w219 w222]
              tunnel: w210 -> [_ w231]
              tunnel: [w219 w228] -> w209
              tunnel: w208 -> [_ w224]
              tunnel: w207 -> [_ w223]
              frame False {
              }
              frame True {
                n95 = call "lsl destroy outlet.vi"("error in (no error)"=w222, "outlet"=w224) -> ("error out"=w225:errorcluster)  [unwired: 9 in]
                n96 = call "lsl destroy outlet.vi"("error in (no error)"=w222, "outlet"=w232) -> ("error out"=w236:errorcluster)  [unwired: 9 in]
                n97 = call "lsl destroy streaminfo.vi"("error in (no error)"=w225, "streaminfo"=w223) -> ("error out"=w221:errorcluster)  [unwired: 9 in]
                n98 = call "lsl destroy streaminfo.vi"("error in (no error)"=w236, "streaminfo"=w231) -> ("error out"=w229:errorcluster)  [unwired: 9 in]
                n99 = call <vilib>:"Clear Errors.vi"("error in (no error)"=w221) -> ()  [unwired: 5 in, 2 out]
                n100 = call <vilib>:"Clear Errors.vi"("error in (no error)"=w229) -> ("error out"=w228:errorcluster)  [unwired: 5 in, 1 out]
                n101 = Bundle By Name(cluster=w235, "LSL Streaming"=FALSE, "Status"="Stoped Stream ...", "Data Chunk.counter"=u8 0 ("Data Chunk .counter"), "Data Chunk.Data"=dbl[][] [] ("Data Chunk .Data")) -> (w234:T3)
              }
            }
          }
          frame "LSL Stream Data" {
            # "1. Gets WiBCI Data and build data Chunk for transfer\n2. Prepare Data for LSL\n3. Broadcast Data"
            n102 = Variant To Data(error in=w249, type=T12 {"WiBCI16T Data"={"EEG Ch 1"=0.0, "EEG Ch 2"=0.0, "EEG Ch 3"=0.0, "EEG Ch 4"=0.0, "EEG Ch 5"=0.0, "EEG Ch 6"=0.0, "EEG Ch 7"=0.0, "EEG Ch 8"=0.0, "EEG Ch 9"=0.0, "EEG Ch 10"=0.0, "EEG Ch 11"=0.0, "EEG Ch 12"=0.0, "EEG Ch 13"=0.0, "EEG Ch 14"=0.0, "EEG Ch 15"=0.0, "EEG Ch 16"=0.0, "X-Accel"=0, "Y-Accel"=0, "Z-Accel"=0, "X-Gyro"=0, "Y-Gyro"=0, "Z-Gyro"=0, "Timer"=0, "Packet ID"=0, "HW Trig1"=0, "SW Trig1"=0, "HW Trig2"=0, "SW Trig2"=0, "WiBCI Status"={"Mode Byte"=0, "Ch Config"=0, "Ch Ref Map"=0, "Ch Enable Map"=0, "Temperature"=0.0, "Battery"=0, "Version"=""}, "Reg Map"={"ADS1"=[], "ADS2"=[]}}} ("LSL Stream Data Argument"), Variant=w248) -> (data=w246:T12, error out=w244:errorcluster)
            n103 = Unbundle By Name(w237) -> ("outlet"=w245:T5, "LSL Streaming"=w242:bool, "Data Chunk"=w241:cluster{"counter":u8, "Data":dbl[][]})
            n104 = case shown="True" w242 {
              tunnel: w246 -> [_ w263]
              tunnel: w245 -> [_ w262]
              tunnel: w244 -> [w253 w261]
              tunnel: [w253 w260] -> w243
              tunnel: w241 -> [w252 w259]
              tunnel: [w251 w257] -> w239
              tunnel: [w250 w255] -> w238
              tunnel: w237 -> [_ w254]
              frame False {
                n105 = Unbundle By Name(w252) -> ("counter"=w251:u8, "Data"=w250:dbl[][])
              }
              frame True {
                n106 = Unbundle By Name(w259) -> ("Data"=w256:dbl[][], "counter"=w258:u8)
                n107 = case shown="0, Default" w258 {
                  selector: w258 -> [w267 w277]
                  tunnel: w263 -> [w270 w285]
                  tunnel: w262 -> [_ w284]
                  tunnel: w261 -> [w269 w282]
                  tunnel: [w269 w281] -> w260
                  tunnel: [w272 u8 0] -> w257
                  tunnel: w256 -> [w268 w279]
                  tunnel: [w265 dbl[][] [] ("Data Chunk .Data")] -> w255
                  tunnel: w254 -> [w264 w274]
                  frame 0, Default {
                    n108 = Unbundle By Name(w270) -> ("WiBCI16T Data"=w271:T13)
                    n109 = call "Prepare Data for LSL.vi"("Data Cluster"=w264, "WiBCI16T Data"=w271) -> ("Prepared Data Array"=w266:dbl[][])  [unwired: 8 in, 1 out]
                    n110 = Insert Into Array(array=w268, index (row)=w267, new element=w266) -> (w265:dbl[][])  [unwired: 1 in]
                    n111 = Increment(x=w267) -> (x+1=w272:u8)
                  }
                  frame 9 {
                    n112 = Unbundle By Name(w285) -> ("WiBCI16T Data"=w283:T13)
                    n113 = call "Prepare Data for LSL.vi"("Data Cluster"=w274, "WiBCI16T Data"=w283) -> ("Data Chunk Size"=w273:i32, "Prepared Data Array"=w278:dbl[][])  [unwired: 8 in]
                    n114 = Insert Into Array(array=w279, index (row)=w277, new element=w278) -> (w276:dbl[][])  [unwired: 1 in]
                    n115 = call "lsl push chunk d.vi"("error in (no error)"=w282, "data_elements"=w273, "data"=w276, "outlet"=w284) -> ("error out"=w281:errorcluster)  [unwired: 6 in, 1 out]
                  }
                }
              }
            }
            n116 = Bundle By Name(cluster=w237, "Data Chunk.counter"=w239, "Data Chunk.Data"=w238) -> (w240:T3)
          }
          frame "Get Listeners count" {
            # "Gets the number of listeners for the LSL"
            n117 = Variant To Data(error in=w300, type=T16 {"Wait Notifier"=refnum, "wait for reply"=FALSE} ("Get Listeners count Argument"), Variant=w299) -> (data=w297:T16, error out=w289:errorcluster)
            n118 = Unbundle By Name(w297) -> ("Wait Notifier"=w296:refnum<notifier>, "wait for reply"=w295:bool)
            n119 = Unbundle By Name(w291) -> ("outlet"=w290:T5, "LSL Streaming"=w286:bool)
            n120 = case shown="False" w286 {
              tunnel: w290 -> [_ w306]
              tunnel: w289 -> [w302 w305]
              tunnel: [0 ("Have Consumers") w304] -> w288
              tunnel: [w302 w303] -> w287
              frame False {
              }
              frame True {
                n121 = call "lsl have consumers.vi"("error in (no error)"=w305, "outlet"=w306) -> ("error out"=w303:errorcluster, "Have Consumers"=w304:i32)  [unwired: 8 in]
              }
            }
            n122 = Bundle By Name(cluster=T20 {"Listeners"=0, "error"={"status"=FALSE, "code"=0, "source"=""}} ("Get Listeners count (Reply Payload)"), "Listeners"=w288, "error"=w287) -> (w294:T20)
            n123 = Merge Errors(w289, w287) -> (w292:errorcluster)
            n124 = case "DQMH_FIRE_NOTIFIER" shown="True" w295 {
              tunnel: w296 -> [_ w308]
              tunnel: w294 -> [_ w307]
              frame False {
              }
              frame True {
                n125 = Send Notification(notification=w307, notifier=w308) -> ()  [unwired: 1 in, 2 out]
              }
            }
          }
          frame "KeyBoard Trigger" {
            # "Sends KeyBoard Trigger to Marker Stream"
            n126 = Variant To Data(error in=w318, type=T17 {"Keyboard Trig"=0} ("KeyBoard Trigger Argument"), Variant=w317) -> (data=w315:T17, error out=w310:errorcluster)
            n127 = Unbundle By Name(w315) -> ("Keyboard Trig"=w313:i16)
            n128 = Unbundle By Name(w314) -> ("LSL Streaming"=w312:bool, "outlet mark"=w311:T5)
            n129 = case shown="True" w312 {
              tunnel: w313 -> [_ w322]
              tunnel: w311 -> [_ w324]
              tunnel: w310 -> [w319 w323]
              tunnel: [w319 w320] -> w309
              frame False {
              }
              frame True {
                n130 = Build Array(w322) -> (w321:i16[])
                n131 = call "lsl push sample d.vi"("error in (no error)"=w323, "data"=w321, "outlet"=w324) -> ("error out"=w320:errorcluster)  [unwired: 7 in, 1 out]
              }
            }
          }
          frame "---Copy This Frame---" {
            # "Duplicate this frame when creating new messages.  Change this comment in the duplicated frame to describe this message."
            n132 = Merge Errors(w327) -> (w326:errorcluster)
          }
          frame "---Exit and Error Handling---" {
            # "Separator - The following cases handle errors and exit messages."
          }
          frame "Simulate MHL Error" {
            # "#DQMH_HowTo The 'Simulate MHL Error' button  illustrates how the MHL handles errors. This event is instructional in nature and can be removed."
            # "Simulate an error occurring at the MHL"
            n133 = call "Module Name--constant.vi"() -> ("Module Name"=w331:string)  [unwired: 11 in]
            n134 = Format Into String(format string="Simulated error originating at Message Handling Loop in %s", w331) -> (resulting string=w332:string)  [unwired: 2 in, 1 out]
            n135 = call <vilib>:"Error Cluster From Error Code.vi"("show call chain? (False)"=TRUE, "error message (\"\")"=w332, "error code (0)"=5001) -> ("error out"=w336:errorcluster)  [unwired: 6 in]
            n136 = Merge Errors(w338, w336) -> (w337:errorcluster)
          }
          frame "Error" {
            # "#CodeRecommended - If the module is running in standalone mode (External Launch = FALSE), this code will pop up an error dialog and call the 'Exit' message if an error occurs. Add more fine-grained error management here."
            # "Error - Check the error message data and respond accordingly. This message is sent by the \"Error Handler\" VIs at the end of each loop in this application."
            n137 = property class="Module Admin"(reference=w341) -> ("Accessors:External Launch"=w340:bool)  [unwired: 1 in, 2 out]
            n138 = Variant To Data(error in=w349, type=errorcluster {"status"=FALSE, "code"=0, "source"=""} ("error constant"), Variant=w343) -> (data=w339:errorcluster, error out=w347:errorcluster)
            n139 = local write "error out"(w339) -> ()
            n140 = call "Error Reported.vi"("Error"=w339) -> ()  [unwired: 10 in, 1 out]
            n141 = case shown="False" w340 {
              tunnel: [w354 _] -> w346
              tunnel: w342 -> [w352 _]
              tunnel: w339 -> [w353 _]
              frame False {
                n142 = disable-structure shown="Default" {
                  disable-tunnel: w353 -> [w355 _]
                  frame condition #0 (active) {
                    # "If the module is running standalone, then pop up an error dialog and call the \"Exit\" message."
                    n143 = call <vilib>:"Simple Error Handler.vi"("error in (no error)"=w355) -> ()  [unwired: 4 in, 5 out]
                  }
                  frame condition #1 {
                    # "To prevent the Simple Error Handler VI from being loaded (e.g. when deploying to a Real-Time target), add the Conditional Disable Symbol \"DQMH_Disable_SEH\" to your project and set it to TRUE."
                  }
                }
                n144 = call-poly <vilib>:"Delacor_lib_QMH_Enqueue Message (poly).vi"("Priority Message? (F)"=TRUE, "Message"="Exit", "Message Queue in"=w352) -> ("error out"=w354:errorcluster)  [unwired: 7 in, 1 out]
              }
              frame True {
                # "If the module was launched externally, calling the Error Reported broadcast VI is the only action performed by the \"Error\" message. The module's caller can then process the error appropriately."
              }
            }
            n145 = Merge Errors(w347, w346) -> (w345:errorcluster)
          }
          frame "Exit" {
            w362 = 91  # 91: not all Exit messages will have an argument
            w364 = TRUE  # Stop the VI
            # "Release the message queue reference"
            # "Exit - Exit the application."
            n146 = Variant To Data(error in=w372, type=T9 {"Origin"="", "Exit via Stop Module Req?"=FALSE, "Wait for Module to stop?"=FALSE} ("Stop Argument"), Variant=w363) -> (data=w360:T9, error out=w369:errorcluster)
            n147 = call <vilib>:"Clear Errors.vi"("error in (no error)"=w369, "specific error code to clear (0: all)"=w362) -> ("error out"=w371:errorcluster)  [unwired: 4 in, 1 out]
            n148 = control-ref of="This VI"() -> (w359:refnum<vi>)
            n149 = call-dynamic "Delacor_lib_QMH_Release Message Queue.vi"("error in"=w371, "Message Queue"=w366) -> ("error out"=w370:errorcluster)  [unwired: 9 in]
            n150 = call "Handle Exit.vi"("Stop Argument"=w360, "Admin in"=w358, "VI reference"=w359) -> ("error out"=w368:errorcluster)  [unwired: 7 in, 1 out]
            n151 = Merge Errors(w370, w368) -> (w367:errorcluster)
            n152 = call "Error Reported.vi"("Error"=w367) -> ()  [unwired: 10 in, 1 out]
            n153 = call "Module Name--constant.vi"() -> ("Module Name"=w357:string)  [unwired: 11 in]
            n154 = case shown="False" w356 {
              tunnel: w357 -> [w373 _]
              frame False {
                n155 = call "Stop Module.vi"("Wait for Module to Stop? (F)"=TRUE, "Origin"=w373) -> ()  [unwired: 9 in, 1 out]
              }
              frame True {
              }
            }
          }
          frame Default {
            # "'Default' case only runs if there is a message that isn't defined in any of the other cases.  Output a programming error."
            n156 = call "Module Name--constant.vi"() -> ("Module Name"=w379:string)  [unwired: 11 in]
            n157 = Format Into String(format string="The invalid message string \"%s\" was received in the Message Handling Loop for module \"%s\".", w380, w379) -> (resulting string=w375:string)  [unwired: 2 in, 1 out]
            n158 = call <vilib>:"Error Cluster From Error Code.vi"("show call chain? (False)"=TRUE, "error message (\"\")"=w375, "error code (0)"=1) -> ("error out"=w382:errorcluster)  [unwired: 6 in]
            n159 = Merge Errors(w383, w382) -> (w384:errorcluster)
          }
        }
        n160 = call-dynamic "Delacor_lib_QMH_Error Handler - Message Handling Loop.vi"("error in"=w130, "Message Queue in"=w119) -> ("dup error in"=w127:errorcluster)  [unwired: 8 in, 1 out]
      }
    }
    frame Error {
      # "Synchronize Caller Events.vi will inform Start Module.vi that the module has launched and will let the code calling Start Module.vi register for broadcasts and would permit the caller receive the broadcast that an error occurred at launch time."
      n161 = call-dynamic "Delacor_lib_QMH_Release Message Queue.vi"("error in"=w392, "Message Queue"=w385) -> ("error out"=w391:errorcluster)  [unwired: 9 in]
      n162 = call "Synchronize Caller Events.vi"("Singleton Module Admin in"=w386) -> ("error out"=w393:errorcluster)  [unwired: 9 in, 1 out]
      n163 = call "Module Name--constant.vi"() -> ("Module Name"=w389:string)  [unwired: 11 in]
      n164 = Format Into String(format string="An error occurred during initialization. %s is no longer running.", w389) -> (resulting string=w387:string)  [unwired: 2 in, 1 out]
      n165 = Merge Errors(w391, w393) -> (w394:errorcluster)
      n166 = call "Error Reported.vi"("Additional Information"=w387, "Error"=w394) -> ()  [unwired: 9 in, 1 out]
    }
  }
  n167 = Merge Errors(w19, w22) -> (w18:errorcluster)
  n168 = call "Close Module.vi"("error in"=w18, "Module Admin in"=w14) -> ("error out"=w20:errorcluster, "External Launch"=w7:bool, "Module Admin out"=w8:refnum<class "Delacor_lib_QMH_Module Admin.lvclass">)  [unwired: 7 in]
  n169 = Unregister For Events(event registration refnum=w13, error in=w20) -> (error out=w17:errorcluster)
  "error out" <- w17
  n170 = case "External Launch?" shown="True" w7 {
    tunnel: w17 -> [_ w395]
    frame False {
    }
    frame True {
      n171 = case shown="No Error" w395 {
        frame No Error {
          n172 = invoke class="VI" method="FP.Close"() -> ()  [unwired: 3 in, 3 out]
        }
        frame Error {
          n173 = invoke class="VI" method="FP.Open"("Activate"=TRUE ("Activate?")) -> ()  [unwired: 4 in, 5 out]
        }
      }
    }
  }
  n174 = local write "Module Admin"(w8) -> ()
